vi "Get Themometer ID.vi"(0 "Initial string":string) -> (1 "Byte Stream File Refnum":refnum<file>, 2 "String W/ ID":string)   [LabVIEW 2020]
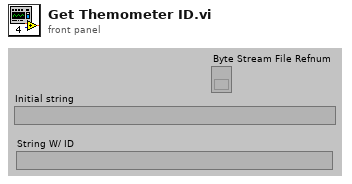
[diagram p1: front panel]
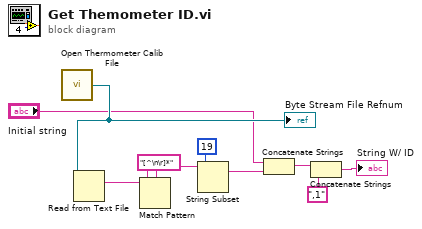
[diagram p0: block diagram]
diagram:
  n1 = call "Open Thermometer Calib File.vi"() -> ("Byte Stream File Refnum"=w10:refnum<file>)
  "Byte Stream File Refnum" <- w10
  n2 = Read from Text File(file (use dialog)=w10) -> (text=w3:string)  [unwired: 3 in, 3 out]
  n3 = Match Pattern(string=w3, regular expression="[^\n\r]*") -> (match substring=w5:string)  [unwired: 1 in, 3 out]
  n4 = String Subset(string=w5, length (rest)=19) -> (substring=w2:string)  [unwired: 1 in]
  n5 = Concatenate Strings("Initial string", w2) -> (w6:string)
  n6 = Concatenate Strings(w6, ",1") -> (→"String W/ ID":string)
